vi "Untitled 1.vi"() -> ()   [LabVIEW 2017]
uses:
  <vilib>/ptbypt/NI_PtbyPt.lvlib
  <vilib>/addons/control/pid/NI_PID_pid.lvlib
  <vilib>/addons/control/pid/pid.llb/PID (DBL).vi
panel:
  out "Array 3":dbl[](array[numeric])
  out "Array 2":dbl[](array[numeric])
  out "Array":u32[](array[numeric])
  out "Numeric 3":i32
  out "x-y":dbl
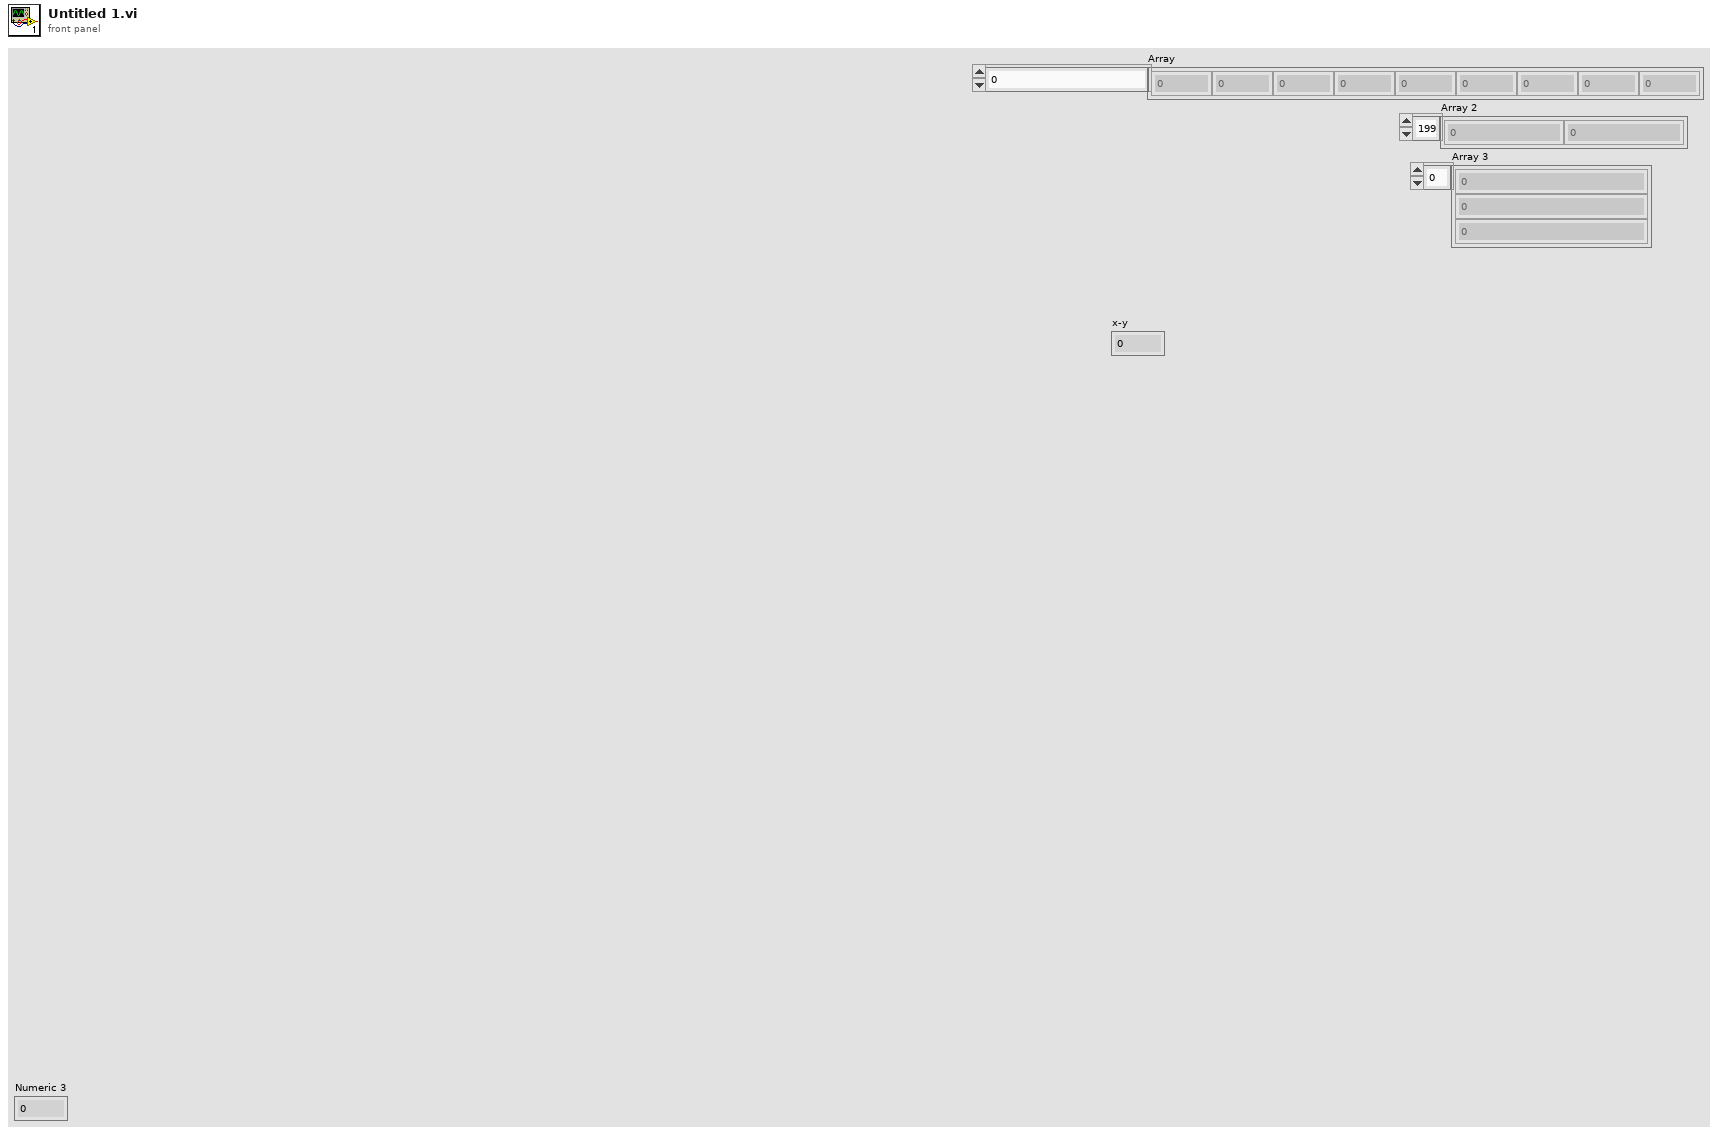
[diagram p1: front panel]
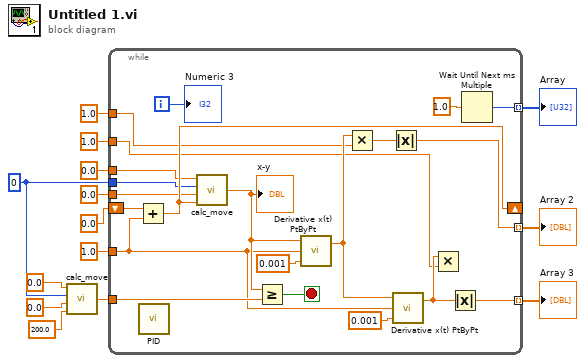
[diagram p0: block diagram]
diagram:
  w1 = 0
  n1 = call "calc_move.vi"("z"=200.0, "y"=0.0, "Numeric"=w1, "x"=0.0) -> ("x-y"=w11:dbl)
  n2 = while {
    shift-right: [w34] -> _
    shift-left: 0.0 -> [w27]
    tunnel: w11 -> [w29]
    tunnel: 1.0 -> [w28]
    tunnel: [w22] -> w8 mode=indexing
    tunnel: 0.0 ("x") -> [w25]
    tunnel: 0.0 ("y") -> [w24]
    tunnel: 1.0 ("y") -> [w21]
    tunnel: 1.0 ("y") -> [w20]
    tunnel: [w19] -> w3 mode=indexing
    tunnel: [w18] -> w2 mode=indexing
    tunnel: w1 -> [w15]
    i -> [w35]
    stop <- w26 stop-if-true
    n3 = Add(x=w27, y=w28) -> (x+y=w34:dbl)
    n4 = call-poly <vilib>:"PID.vi"() -> ()  [unwired: 10 in, 2 out]
    n5 = call "calc_move.vi"("z"=w34, "y"=w24, "Numeric"=w15, "x"=w25) -> ("x-y"=w30:dbl)
    "x-y" <- w30
    n6 = Greater Or Equal?(x=w30, y=w29) -> (x >= y?=w26:bool)
    n7 = call <vilib>:"Derivative x(t) PtByPt.vi"("dt"=0.001, "initial condition"=w28, "x"=w30) -> ("dx/dt"=w33:dbl)  [unwired: 1 in, 1 out]
    n8 = Multiply(x=w33, y=w21) -> (x*y=w32:dbl)
    n9 = Absolute Value(x=w32) -> (abs(x)=w19:dbl)
    n10 = call <vilib>:"Derivative x(t) PtByPt.vi"("dt"=0.001, "initial condition"=w28, "x"=w33) -> ("dx/dt"=w31:dbl)  [unwired: 1 in, 1 out]
    n11 = Multiply(x=w31, y=w20) -> ()  [unwired: 1 out]
    n12 = Absolute Value(x=w31) -> (abs(x)=w18:dbl)
    n13 = Wait Until Next ms Multiple(millisecond multiple=sgl 1.0) -> (millisecond timer value=w22:u32)
    "Numeric 3" <- w35
  }
  "Array" <- w8
  "Array 2" <- w3
  "Array 3" <- w2
